vi "Load Parameters.vi"(8 "error in (no error)":errorcluster, 10 "Resource":variant, 11 "Analyze Actor in":refnum<class "Analyze Actor.lvclass">) -> (0 "error out":errorcluster, 3 "Analyze Actor out":refnum<class "Analyze Actor.lvclass">)   [LabVIEW 2014, in "Analyze Actor.lvlib" / "Analyze Actor.lvclass"]
uses:
  Analyze Actor.lvclass
  Analyze Actor.lvclass/Analyze Actor.ctl
  Analyze Classes/Analyze BaseClass/Analyze BaseClass/Analyze BaseClass.lvclass
  <vilib>/Utility/config.llb/NI_LVConfig.lvlib
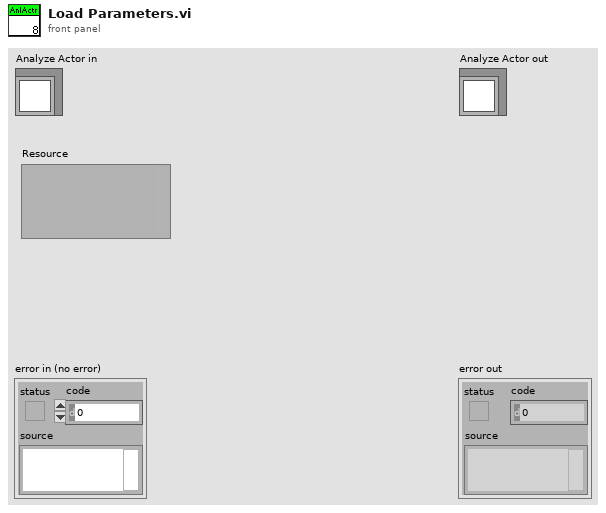
[diagram p1: front panel]
types:
  T1 = typedef "NI_LVConfig.lvlib/Config Data RefNum.ctl" = refnum<k1>
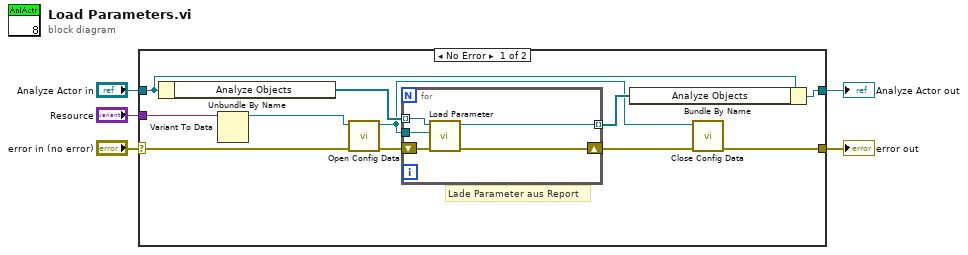
[diagram p0: block diagram]
diagram:
  n1 = case shown="No Error" "error in (no error)" {
    selector: "error in (no error)" -> [w12 w23]
    tunnel: [w9 w23] -> w4
    tunnel: [w14 w22] -> w2
    tunnel: "Analyze Actor in" -> [w16 w22]
    tunnel: "Resource" -> [w8 _]
    frame No Error {
      # "Lade Parameter aus Report"
      n2 = Unbundle By Name(w16) -> ("Analyze Objects"=w15:refnum<class "Analyze BaseClass.lvclass">[])
      n3 = Variant To Data(Variant=w8) -> (data=w7:path)  [unwired: 2 in, 1 out]
      n4 = call <vilib>:"Open Config Data.vi"("error in (no error)"=w12, "configuration file path"=w7) -> ("error out"=w11:errorcluster, "refnum"=w6:T1)  [unwired: 7 in, 1 out]
      n5 = for {
        tunnel: w15 -> [w21] mode=indexing
        tunnel: w6 -> [w20]
        shift-right: [w18] -> w10
        shift-left: w11 -> [w19]
        tunnel: [w17] -> w13 mode=indexing
        n6 = call-dynamic "Load Parameter.vi"("error in (no error)"=w19, "Resource"=w20, "Analyze BaseClass in"=w21) -> ("error out"=w18:errorcluster, "Analyze BaseClass out"=w17:refnum<class "Analyze BaseClass.lvclass">)  [unwired: 7 in]
      }
      n7 = Bundle By Name(cluster=w16, "Analyze Objects"=w13) -> (w14:refnum<class "Analyze Actor.lvclass">)
      n8 = call <vilib>:"Close Config Data.vi"("error in (no error)"=w10, "refnum"=w6) -> ("error out"=w9:errorcluster)  [unwired: 8 in, 1 out]
    }
    frame Error {
    }
  }
  "error out" <- w4
  "Analyze Actor out" <- w2
